vi "Calculate Group Status.vi"(1 "Test Statii":T1[](array[typedef])) -> (0 "Group Status":T1)   [LabVIEW 2011]
uses:
  Test Status.ctl
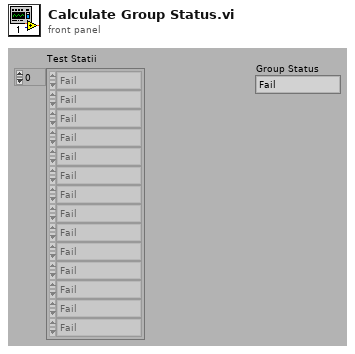
[diagram p1: front panel]
types:
  T1 = typedef "Test Status.ctl" = enum16{"Fail", "Pass", "Abort", "Error", "Done", "Pass by Sample", "Fail by Sample", "Pass Override", "Fail Override", "Not Tested"}
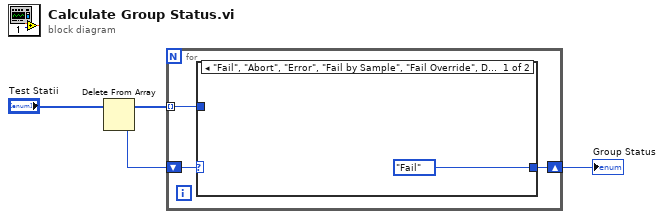
[diagram p0: block diagram]
diagram:
  n1 = Delete From Array(array="Test Statii") -> (deleted portion=w3:T1, array with subset deleted=w2:T1[])  [unwired: 2 in]
  n2 = for {
    shift-right: [w5] -> w1
    shift-left: w3 -> [w7]
    tunnel: w2 -> [w6] mode=indexing
    n3 = case shown="\"Fail\", \"Abort\", \"Error\", \"Fail by Sample\", \"Fail Override\", Default" w7 {
      tunnel: w6 -> [_ w9]
      tunnel: [Test_Status."Fail" ("Group Status") w9] -> w5
      frame "Fail", "Abort", "Error", "Fail by Sample", "Fail Override", Default {
      }
      frame "Pass", "Done", "Pass by Sample", "Pass Override", "Not Tested" {
      }
    }
  }
  "Group Status" <- w1
